vi "GDSIconEditor_TerminaLayoutWindow.vi"(10 "ViRef":refnum<vi>, 11 "ControlQueue":refnum<queue>) -> ()   [LabVIEW 2020]
uses:
  <vilib>/Utility/miscctls.llb/LVRectTypeDef.ctl
panel:
  out "LayoutPicture":picture
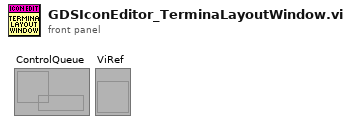
[diagram p1: front panel]
types:
  T1 = typedef "LVRectTypeDef.ctl" = cluster{"Left":i16, "Top":i16, "Right":i16, "Bottom":i16}
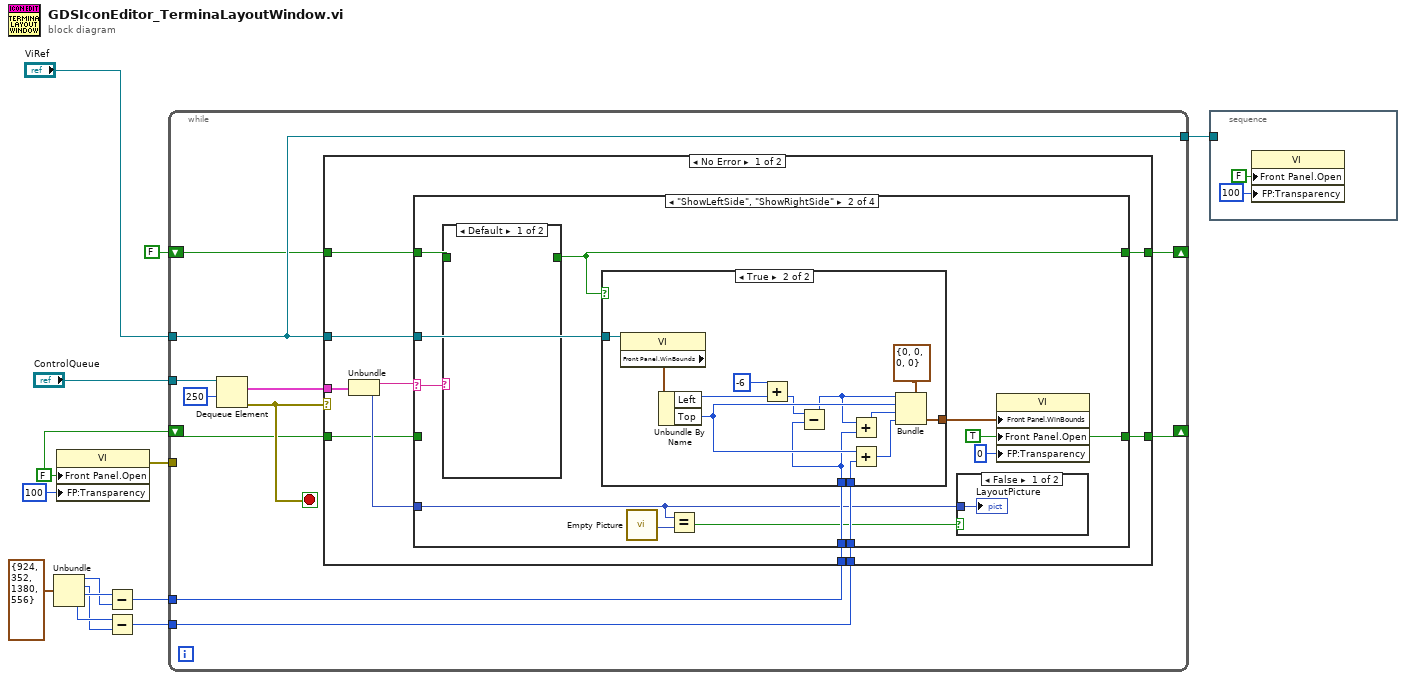
[diagram p0: block diagram]
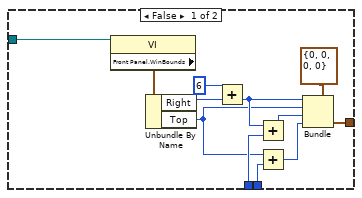
[diagram p4: hidden frame]
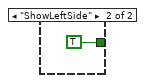
[diagram p5: hidden frame]
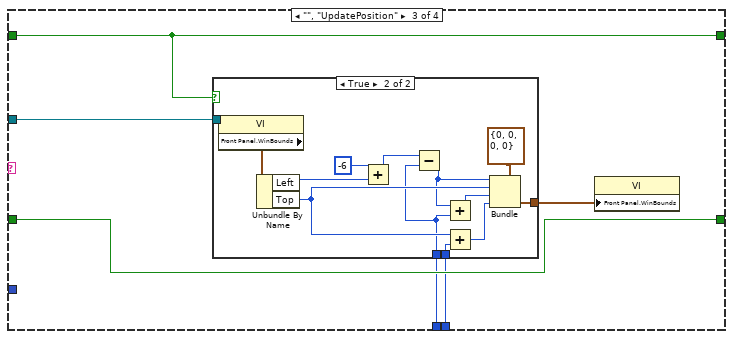
[diagram p6: hidden frame]
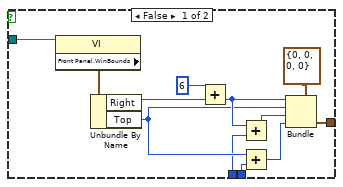
[diagram p7: hidden frame]
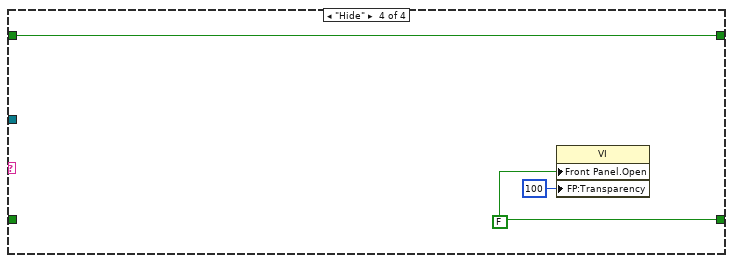
[diagram p8: hidden frame]
diagram:
  w2 = FALSE ("Front Panel Window:Open")
  n1 = Unbundle(T1 {"Left"=924, "Top"=352, "Right"=1380, "Bottom"=556} ("Front Panel Window:Window Bounds")) -> ("Left"=w10:i16, "Top"=w8:i16, "Right"=w11:i16, "Bottom"=w9:i16)
  n2 = property class="VI"("Front Panel.Open"=w2, "FP:Transparency"=u8 100 ("Front Panel Window:Transparency")) -> (error out=w4:errorcluster)  [unwired: 2 in, 1 out]
  n3 = Subtract(x=w11, y=w10) -> (x-y=w7:i16)
  n4 = Subtract(x=w9, y=w8) -> (x-y=w6:i16)
  n5 = while {
    tunnel: "ControlQueue" -> [w25]
    tunnel: "ViRef" -> [w20]
    tunnel: w7 -> [w22]
    tunnel: w6 -> [w21]
    tunnel: [w20] -> w5
    tunnel: w4 -> [_]
    shift-right: [w19] -> _
    shift-left: w2 -> [w18]
    shift-right: [w15] -> _
    shift-left: FALSE -> [w16]
    stop <- w23 stop-if-true
    n6 = Dequeue Element(queue=w25, timeout in ms (-1)=250) -> (element=w24:cluster{"Message":string, "Picture":picture}, error out=w23:errorcluster)  [unwired: 1 in, 2 out]
    n7 = case shown="No Error" w23 {
      tunnel: w24 -> [w32 _]
      tunnel: w20 -> [w35 _]
      tunnel: w22 -> [w34 _]
      tunnel: w21 -> [w33 _]
      tunnel: [w29 _] -> w19
      tunnel: w18 -> [w28 _]
      tunnel: w16 -> [w27 w111]
      tunnel: [w26 w111] -> w15
      frame No Error {
        n8 = Unbundle(w32) -> ("Message"=w31:string, "Picture"=w30:picture)
        n9 = case shown="\"ShowLeftSide\", \"ShowRightSide\"" w31 {
          selector: w31 -> [_ w43 _ _]
          tunnel: w35 -> [_ w49 w81 _]
          tunnel: w34 -> [_ w48 w79 _]
          tunnel: w33 -> [_ w47 w78 _]
          tunnel: w30 -> [_ w39 _ _]
          tunnel: [w37 w44 w80 w109] -> w29
          tunnel: w28 -> [w37 _ w80 _]
          tunnel: w27 -> [w36 w42 w77 w108]
          tunnel: [w36 w41 w77 w108] -> w26
          frame Default {
          }
          frame "ShowLeftSide", "ShowRightSide" {
            w44 = TRUE ("Front Panel Window:Open")
            n10 = case shown="Default" w43 {
              tunnel: w42 -> [_ _]
              tunnel: [_ TRUE] -> w41
              frame Default {
              }
              frame "ShowLeftSide" {
              }
            }
            n11 = case shown="True" w41 {
              tunnel: w49 -> [w62 w75]
              tunnel: w48 -> [w55 w65]
              tunnel: w47 -> [w53 w68]
              tunnel: [w51 w66] -> w46
              frame False {
                n12 = property class="VI"(reference=w62) -> ("Front Panel.WinBounds"=w61:T1)  [unwired: 1 in, 2 out]
                n13 = Unbundle By Name(w61) -> ("Right"=w60:i16, "Top"=w54:i16)
                n14 = Add(x=i16 6, y=w60) -> (x+y=w57:i16)
                n15 = Add(x=w57, y=w55) -> (x+y=w56:i16)
                n16 = Add(x=w54, y=w53) -> (x+y=w52:i16)
                n17 = Bundle(cluster=T1 {"Left"=0, "Top"=0, "Right"=0, "Bottom"=0} ("Front Panel Window:Window Bounds"), "Left"=w57, "Top"=w54, "Right"=w56, "Bottom"=w52) -> (w51:T1)
              }
              frame True {
                n18 = property class="VI"(reference=w75) -> ("Front Panel.WinBounds"=w74:T1)  [unwired: 1 in, 2 out]
                n19 = Unbundle By Name(w74) -> ("Left"=w73:i16, "Top"=w69:i16)
                n20 = Add(x=i16 -6, y=w73) -> (x+y=w64:i16)
                n21 = Subtract(x=w64, y=w65) -> (x-y=w63:i16)
                n22 = Add(x=w63, y=w65) -> (x+y=w70:i16)
                n23 = Add(x=w69, y=w68) -> (x+y=w67:i16)
                n24 = Bundle(cluster=T1 {"Left"=0, "Top"=0, "Right"=0, "Bottom"=0} ("Front Panel Window:Window Bounds"), "Left"=w63, "Top"=w69, "Right"=w70, "Bottom"=w67) -> (w66:T1)
              }
            }
            n25 = call "Empty Picture"() -> ("empty picture"=w40:picture)
            n26 = Equal?(x=w39, y=w40) -> (x = y?=w38:bool)
            n27 = case shown="False" w38 {
              tunnel: w39 -> [w50 _]
              frame False {
                "LayoutPicture" <- w50
              }
              frame True {
              }
            }
            n28 = property class="VI"("Front Panel.WinBounds"=w46, "Front Panel.Open"=w44, "FP:Transparency"=u8 0 ("Front Panel Window:Transparency")) -> ()  [unwired: 2 in, 2 out]
          }
          frame "", "UpdatePosition" {
            n29 = case shown="True" w77 {
              tunnel: [w86 w100] -> w82
              tunnel: w81 -> [w85 w99]
              tunnel: w79 -> [w84 w97]
              tunnel: w78 -> [w83 w98]
              frame False {
                n30 = property class="VI"(reference=w85) -> ("Front Panel.WinBounds"=w94:T1)  [unwired: 1 in, 2 out]
                n31 = Unbundle By Name(w94) -> ("Right"=w93:i16, "Top"=w88:i16)
                n32 = Add(x=i16 6, y=w93) -> (x+y=w90:i16)
                n33 = Add(x=w90, y=w84) -> (x+y=w89:i16)
                n34 = Add(x=w88, y=w83) -> (x+y=w87:i16)
                n35 = Bundle(cluster=T1 {"Left"=0, "Top"=0, "Right"=0, "Bottom"=0} ("Front Panel Window:Window Bounds"), "Left"=w90, "Top"=w88, "Right"=w89, "Bottom"=w87) -> (w86:T1)
              }
              frame True {
                n36 = property class="VI"(reference=w99) -> ("Front Panel.WinBounds"=w107:T1)  [unwired: 1 in, 2 out]
                n37 = Unbundle By Name(w107) -> ("Left"=w106:i16, "Top"=w102:i16)
                n38 = Add(x=i16 -6, y=w106) -> (x+y=w96:i16)
                n39 = Subtract(x=w96, y=w97) -> (x-y=w95:i16)
                n40 = Add(x=w95, y=w97) -> (x+y=w103:i16)
                n41 = Add(x=w102, y=w98) -> (x+y=w101:i16)
                n42 = Bundle(cluster=T1 {"Left"=0, "Top"=0, "Right"=0, "Bottom"=0} ("Front Panel Window:Window Bounds"), "Left"=w95, "Top"=w102, "Right"=w103, "Bottom"=w101) -> (w100:T1)
              }
            }
            n43 = property class="VI"("Front Panel.WinBounds"=w82) -> ()  [unwired: 2 in, 2 out]
          }
          frame "Hide" {
            w109 = FALSE ("Front Panel Window:Open")
            n44 = property class="VI"("Front Panel.Open"=w109, "FP:Transparency"=u8 100 ("Front Panel Window:Transparency")) -> ()  [unwired: 2 in, 2 out]
          }
        }
      }
      frame Error {
      }
    }
  }
  n45 = stacked-sequence {
    tunnel: w5 -> [_]
    frame #0 {
      n46 = property class="VI"("Front Panel.Open"=FALSE ("Front Panel Window:Open"), "FP:Transparency"=u8 100 ("Front Panel Window:Transparency")) -> ()  [unwired: 2 in, 2 out]
    }
  }
